vi "Configure Named Icons.vi"() -> ()   [LabVIEW 2020]
doc: "Run this VI to configure the text that LabVIEW uses to populate the icon of VIs with abbreviations and ignored words. Enter your desired abbreviations and ignored words into the two arrays then run the VI to save it into the LabVIEW configuration file."
uses:
  <resource>/dialog/lvconfig.llb/LV Config Write String.vi
panel:
  in  "Words to ignore entirely":string[](array[string])
  in  "Words to abbreviate":string[][](array[string])
  # "original"
  # "shortened"
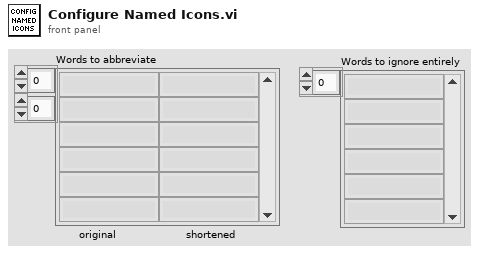
[diagram p1: front panel]
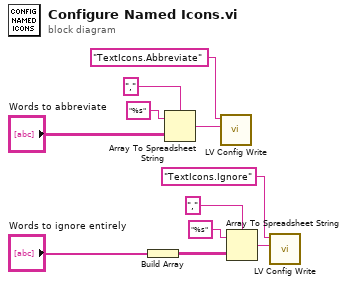
[diagram p0: block diagram]
diagram:
  n1 = Build Array("Words to ignore entirely") -> (w3:string[][])
  n2 = Array To Spreadsheet String(delimiter (Tab)=",", array="Words to abbreviate", 3:"%s" ("format string")) -> (spreadsheet string=w10:string)
  n3 = call-poly <resource>:"LV Config Write.vi"("value"=w10, "key"="TextIcons.Abbreviate" ("section")) -> ()  [unwired: 5 in, 1 out]
  n4 = Array To Spreadsheet String(delimiter (Tab)=",", array=w3, 3:"%s" ("format string")) -> (spreadsheet string=w1:string)
  n5 = call-poly <resource>:"LV Config Write.vi"("value"=w1, "key"="TextIcons.Ignore" ("section")) -> ()  [unwired: 5 in, 1 out]
